vi "Veristand API.vi"() -> ()   [LabVIEW 2019]
uses:
  <vilib>/NI VeriStand/Execution/Workspace/NI VeriStand - Get Single Channel Value.vi
  <vilib>/NI VeriStand/Execution/Workspace/NI_VS Workspace ExecutionAPI.lvlib
panel:
  out "error out":errorcluster
  out "i":i32
  in  "stop":bool
  out "channel name":string
  in  "Channel":i32
  out "Aliases":string[](array[string])
  out "Channels":string[](array[string])
  out "Value":dbl
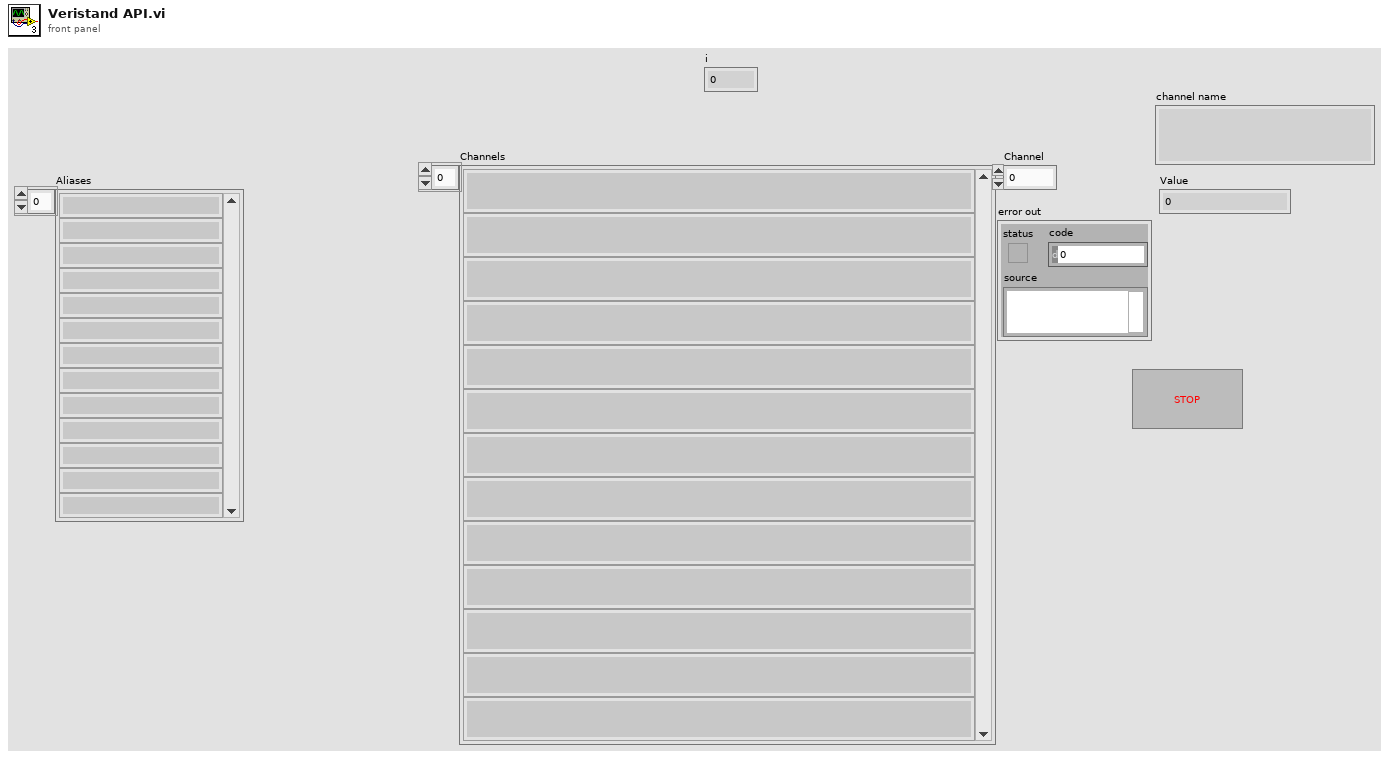
[diagram p1: front panel]
types:
  T1 = typedef "NI_VS Workspace ExecutionAPI.lvlib/WorkspaceAPI.ctl" = refnum<k24>
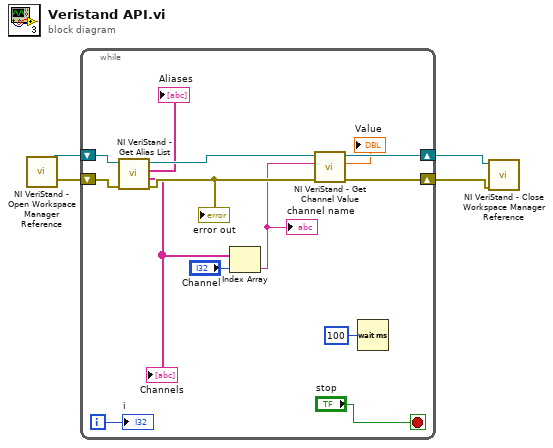
[diagram p0: block diagram]
diagram:
  n1 = call <vilib>:"NI VeriStand - Open Workspace Manager Reference.vi"() -> ("error out"=w1:errorcluster, "WorkspaceManager"=w2:T1)  [unwired: 10 in]
  n2 = while {
    shift-right: [w18] -> w4
    shift-left: w2 -> [w15]
    shift-right: [w17] -> w3
    shift-left: w1 -> [w14]
    i -> [w5]
    stop <- "stop" stop-if-true
    n3 = call <vilib>:"NI VeriStand - Get Alias List.vi"("error in (no error)"=w14, "WorkspaceManager in"=w15) -> ("error out"=w13:errorcluster, "Channels"=w10:string[], "Aliases"=→"Aliases":string[], "WorkspaceManager out"=w12:T1)  [unwired: 6 in]
    "Channels" <- w10
    "error out" <- w13
    n4 = Index Array(array=w10, index="Channel") -> (element=w9:string)
    "channel name" <- w9
    n5 = call-poly <vilib>:"NI VeriStand - Get Channel Value.vi"("error in (no error)"=w13, "Channel"=w9, "WorkspaceManager in"=w12) -> ("error out"=w17:errorcluster, "Value"=→"Value":dbl, "WorkspaceManager out"=w18:T1)  [unwired: 6 in]
    n6 = Wait (ms)(milliseconds to wait=u32 100) -> ()  [unwired: 1 out]
    "i" <- w5
  }
  n7 = call <vilib>:"NI VeriStand - Close Workspace Manager Reference.vi"("error in (no error)"=w3, "WorkspaceManager"=w4) -> ()  [unwired: 9 in, 1 out]
